vi "BASE-User Details.vi"(7 "Enum":enum16{"Read", "Write"}(ring)=enum."Write", 10 "Level In":i32, 11 "User Name In":string) -> (2 "Level Out":i32, 3 "User Name Out":string)   [LabVIEW 2017]
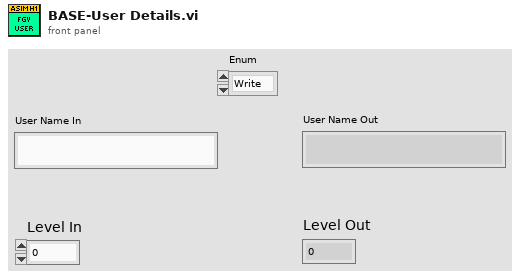
[diagram p1: front panel]
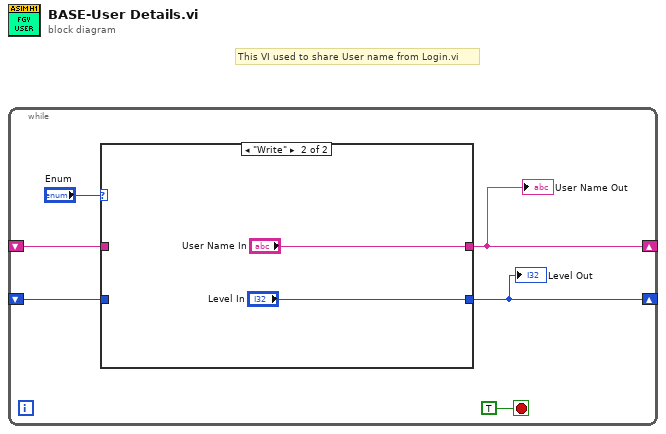
[diagram p0: block diagram]
diagram:
  # "This VI used to share User name from Login.vi"
  n1 = while {
    shift-right: [w3] -> _
    shift-left: _ -> [w4]
    shift-right: [w2] -> _
    shift-left: _ -> [w1]
    stop <- TRUE stop-if-true
    n2 = case shown="\"Write\"" "Enum" {
      tunnel: [w8 "User Name In"] -> w3
      tunnel: w4 -> [w8 _]
      tunnel: [w7 "Level In"] -> w2
      tunnel: w1 -> [w7 _]
      frame "Read", Default {
      }
      frame "Write" {
      }
    }
    "User Name Out" <- w3
    "Level Out" <- w2
  }
